vi "AcqZERO_SARAH.vi"(4 "entrée d'erreur":errorcluster caption="entrée d'erreur (pas d'erreur)", 6 "Fichier":string, 7 "Projet":string) -> (0 "sortie d'erreur":errorcluster)   [LabVIEW 2017]
uses:
  DefDeType/WhichPath.ctl
  <vilib>/DAQmx/read.llb/DAQmx Read (Analog 2D DBL NChan NSamp).vi
  <vilib>/DAQmx/configure/task.llb/DAQmx Configure Logging (TDMS).vi
  <vilib>/DAQmx/miscellaneous.llb/DAQmx Fill In Error Info.vi
panel:
  out "Glissière":i32(slide) scale=0.0..100.0
  out "Graphe déroulant":dbl[][](graph)
  out "fichier :":path
  # "Wave Gauges Zero Acquisition"
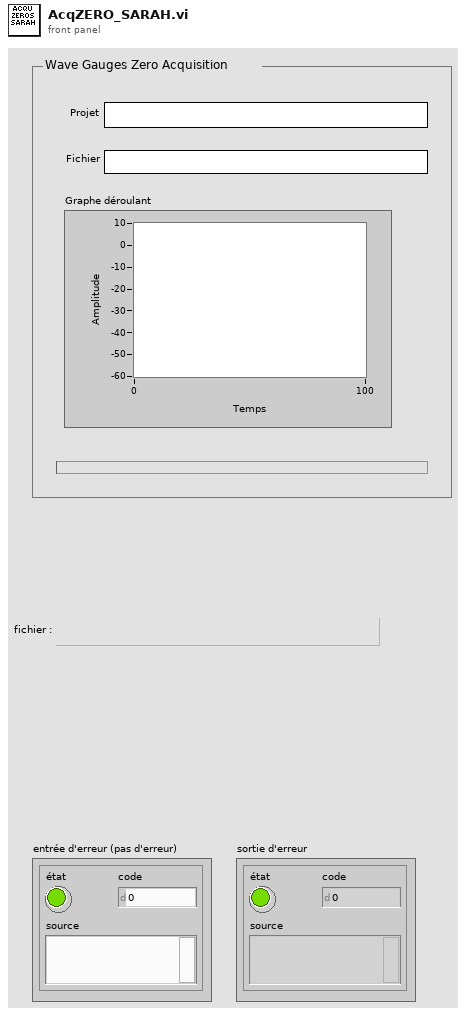
[diagram p1: front panel]
types:
  T1 = typedef "WhichPath.ctl" = enum16{"DossierProjet", "Config", "Meas", "MeasPCI", "MeasCRIO1", "MeasCRIO2", "MeasQualisys", "MeasHBM", "MeasTDMS", "Fig", "Res"}
  T2 = typedef "ConfigTotale.ctl" = cluster{"VoltageChannels":T3, "WheastoneBridgeChannels":T4, "Configuration":T5}
  T3 = typedef "VoltageChannels.ctl" = cluster{"ChannelNames":string[], "Sensitivity(Unit/V)":dbl[], "AutoZero":bool[], "ChannelUnits":string[], "Offsets(Units)":dbl[], "Graph Num":u8[]}
  T4 = typedef "WBridgeChannels.ctl" = cluster{"ChannelNames":string[], "Sensitivity(Unit/V)":dbl[], "AutoZero":bool[], "ChannelUnits":string[], "Offsets(Units)":dbl[], "Graph Num":u8[]}
  T5 = typedef "Configuration.ctl" = cluster{"AcqSamplingRate(Hz)":u32, "AcqTime(s)":u32, "Trigger":bool, "NbVoltageChannels":u32, "NbWBridgeChannels":u32, "Qualisys":bool, "Hexapode":bool, "FinalSamplingRate(Hz)":u32, "QualisysDataType":enum16{"6DOF", "3DTracking", "6DOF + 3D"}, "Nortek":bool, "HBM":bool}
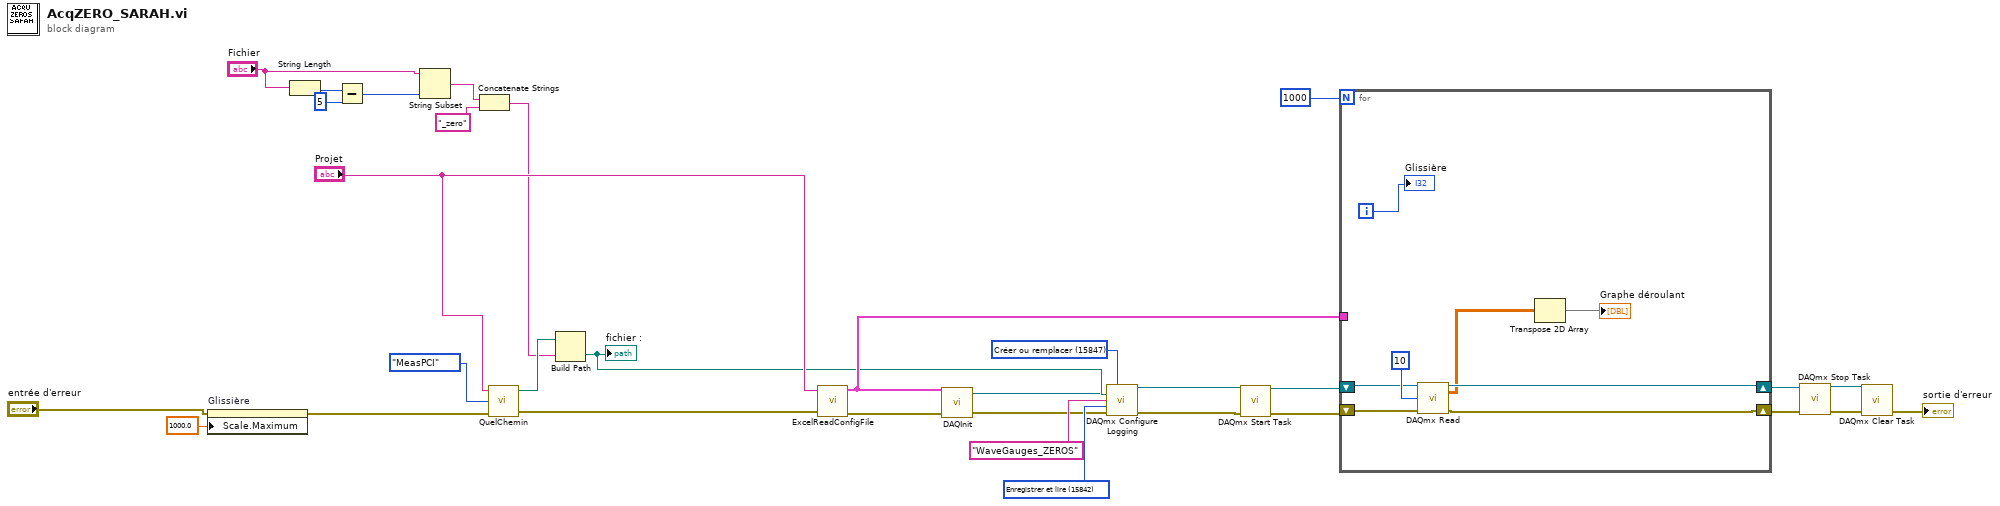
[diagram p0: block diagram]
diagram:
  w4 = 15847 items=["Ouvrir"=10437, "Ouvrir ou créer"=15846, "Créer ou remplacer"=15847, "Créer"=15848] ("operation")
  w11 = 15842 items=["Off"=10231, "Enregistrer"=15844, "Enregistrer et lire"=15842] ("logging mode")
  n1 = property on="Glissière" class="Gliss (strict)"(error in="entrée d'erreur", "Scale.Maximum"=1000.0 ("Échelle.Gamme:Maximum")) -> (error out=w3:errorcluster)  [unwired: 1 in, 1 out]
  n2 = String Length(string="Fichier") -> (length=w22:i32)
  n3 = Subtract(x=w22, y=5) -> (x-y=w20:i32)
  n4 = String Subset(string="Fichier", length (rest)=w20) -> (substring=w18:string)  [unwired: 1 in]
  n5 = Concatenate Strings(w18, "_zero" ("chaîne")) -> (w16:string)
  n6 = call "QuelChemin.vi"("Entrée d'erreur"=w3, "WhichPath?"=WhichPath."MeasPCI", "NomProjet"="Projet") -> ("Sortie d'erreur"=w15:errorcluster, "SurDisqueLocal"=w29:path)  [unwired: 1 out]
  n7 = Build Path(base path=w29, name or relative path=w16) -> (appended path=w13:path)
  "fichier :" <- w13
  n8 = call "ExcelReadConfigFile.vi"("NomProjet"="Projet", "error in (no error)"=w15) -> ("ConfigurationTotale"=w27:T2, "error out"=w28:errorcluster)  [unwired: 3 in]
  n9 = call "DAQInit.vi"("error in"=w28, "configInput"=w27) -> ("error out"=w10:errorcluster, "task out"=w9:refnum<k21>)  [unwired: 2 in]
  n10 = call-poly <vilib>:"DAQmx Configure Logging.vi"("task/channels in"=w9, "operation"=w4, "file path"=w13, "group name"="WaveGauges_ZEROS", "logging mode"=w11, "error in"=w10) -> ("task out"=w8:refnum<k21>, "error out"=w6:errorcluster)  [unwired: 8 in]
  n11 = call <vilib>:"DAQmx Start Task.vi"("task/channels in"=w8, "error in"=w6) -> ("task out"=w7:refnum<k21>, "error out"=w5:errorcluster)  [unwired: 12 in]
  n12 = for {
    N: 1000 ("taille de la dimension") -> [_]
    shift-right: [w36] -> w25
    shift-left: w5 -> [w40]
    tunnel: w27 -> [_]
    shift-right: [w37] -> w26
    shift-left: w7 -> [w38]
    i -> [w33]
    n13 = call-poly <vilib>:"DAQmx Read.vi"("task/channels in"=w38, "number of samples per channel"=10, "error in"=w40) -> ("task out"=w37:refnum<k21>, "data"=w34:dbl[][], "error out"=w36:errorcluster)  [unwired: 10 in]
    n14 = Transpose 2D Array(2D array=w34) -> (transposed array=→"Graphe déroulant":dbl[][])
    "Glissière" <- w33
  }
  n15 = call <vilib>:"DAQmx Stop Task.vi"("task/channels in"=w26, "error in"=w25) -> ("task out"=w23:refnum<k21>, "error out"=w24:errorcluster)  [unwired: 12 in]
  n16 = call <vilib>:"DAQmx Clear Task.vi"("task in"=w23, "error in"=w24) -> ("error out"=→"sortie d'erreur":errorcluster)  [unwired: 13 in]
